vi "Log AI.vi"(8 "error in (no error)":errorcluster, 11 "Instrument.Lockin in":refnum<class "Instrument.Lockin.lvclass">) -> (0 "error out":errorcluster, 3 "Instrument.Lockin out":refnum<class "Instrument.Lockin.lvclass">)   [LabVIEW 2019, in "Instrument.Lockin.lvlib" / "Instrument.Lockin.lvclass"]
uses:
  Instrument.Lockin.lvclass
  C:/Program Files/National Instruments/LabVIEW 2019/user.lib/LevyLab/Instrument Framework/Instrument/Instrument.lvclass
  Instrument.Lockin.lvclass/Instrument.Lockin.ctl
  <userlib>/LevyLab/Instrument Framework/Instrument/Instrument.lvclass
  C:/Program Files/National Instruments/LabVIEW 2019/user.lib/LevyLab/Instrument Framework/Instrument Types/Lockin/Instrument.LockinAPI.lvclass
  C:/Program Files/National Instruments/LabVIEW 2019/vi.lib/JKI/JKI SMO/SMO/SMO.lvclass
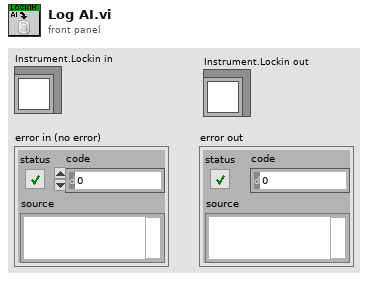
[diagram p1: front panel]
types:
  T1 = typedef "Instrument.Lockin.lvlib/Instrument.Lockin.lvclass/Lockin.LogSweepAOAI--Cluster.ctl" = cluster{"ChassisSerialNumber":u32, "Channel":i32, "Data":dbl, "Sweeping?":bool}
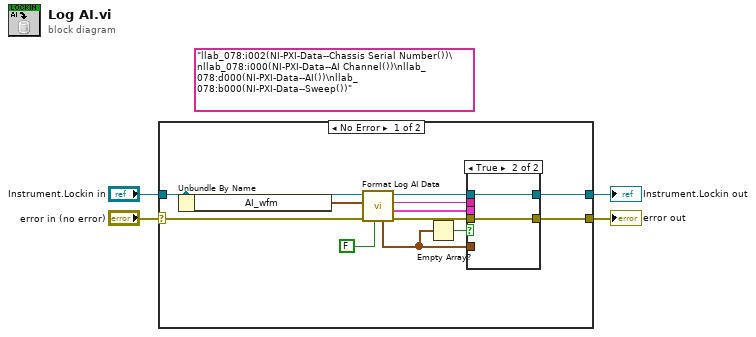
[diagram p0: block diagram]
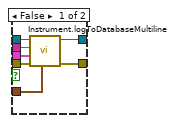
[diagram p2: hidden frame]
diagram:
  (unwired) "llab_078:i002(NI-PXI-Data--Chassis Serial Number())\nllab_078:i000(NI-PXI-Data--AI Channel())\nllab_078:d000(NI-PXI-Data--AI())\nllab_078:b000(NI-PXI-Data--Sweep())"
  n1 = case shown="No Error" "error in (no error)" {
    selector: "error in (no error)" -> [w15 w27]
    tunnel: "Instrument.Lockin in" -> [w14 w26]
    tunnel: [w16 w27] -> w3
    tunnel: [w12 w26] -> w1
    frame No Error {
      n2 = Unbundle By Name(w14) -> ("AI_wfm"=w13:waveform(dbl)[])
      n3 = call "Format Log AI Data.vi"("Sweeping?"=FALSE, "error in (no error)"=w15, "waveform"=w13, "Instrument.Lockin in"=w14) -> ("error out"=w6:errorcluster, "Log Data"=w9:T1[], "Log Paths"=w10:string, "Instrument.Lockin out"=w11:refnum<class "Instrument.Lockin.lvclass">, "Times"=w7:timestamp[])  [unwired: 3 in]
      n4 = Empty Array?(array=w7) -> (empty?=w5:bool)
      n5 = case shown="True" w5 {
        tunnel: [w23 w24] -> w16
        tunnel: w11 -> [w22 w25]
        tunnel: w10 -> [w21 _]
        tunnel: w9 -> [w20 _]
        tunnel: [w19 w25] -> w12
        tunnel: w7 -> [w18 _]
        tunnel: w6 -> [w17 w24]
        frame False {
          n6 = call <userlib>:"Instrument.logToDatabaseMultiline.vi"("timestamps"=w18, "error in (no error)"=w17, "Data"=w20, "Paths"=w21, "Instrument"=w22) -> ("error out"=w23:errorcluster, "Instrument out"=w19:refnum<class "Instrument.Lockin.lvclass">)  [unwired: 5 in]
        }
        frame True {
        }
      }
    }
    frame Error {
    }
  }
  "error out" <- w3
  "Instrument.Lockin out" <- w1
